vi "Write Volts.vi"(8 "error in (no error)":errorcluster, 10 "Volts":dbl min=0.0 step=0.001, 11 "Voltage in":refnum<class "Voltage.lvclass">) -> (0 "error out":errorcluster, 3 "Voltage out":refnum<class "Voltage.lvclass">)   [LabVIEW 2023, in "HAF.lvlib" / "Voltage.lvclass"]
uses:
  Voltage.lvclass
  Voltage.lvclass/Voltage.ctl
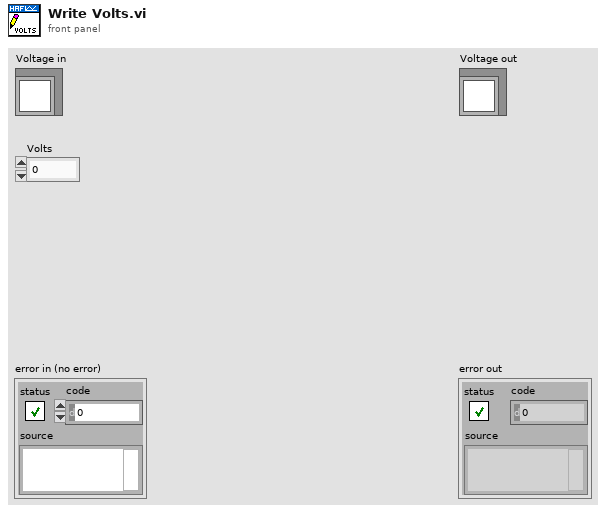
[diagram p1: front panel]
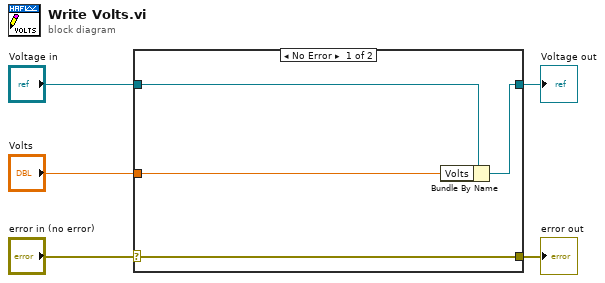
[diagram p0: block diagram]
diagram:
  n1 = case shown="No Error" "error in (no error)" {
    selector: "error in (no error)" -> [w9 w10]
    tunnel: [w9 w10] -> w4
    tunnel: [w7 w11] -> w2
    tunnel: "Voltage in" -> [w8 w11]
    tunnel: "Volts" -> [w6 _]
    frame No Error {
      n2 = Bundle By Name(cluster=w8, "Volts"=w6) -> (w7:refnum<class "Voltage.lvclass">)
    }
    frame Error {
    }
  }
  "error out" <- w4
  "Voltage out" <- w2
